vi "Fix BDPW Checksum.vi"(9 "Terminal Counts":T1, 10 "Only fix 3rd hash (F)":bool, 11 "Resources in":T2) -> (3 "Resources out":T2)   [LabVIEW 2018, in "Resource Manipulation.lvlib"]
uses:
  Resource Manipulation/Resource Array.ctl
  Resource Manipulation/Resource.ctl
  Resource Manipulation/Terminal Counts.ctl
  <userlib>/_OpenG.lib/md5/md5.llb/MD5 Message Digest (Binary String)__ogtk.vi
  Resource Manipulation/Find Resource by Type (String).vi
  Resource Manipulation.lvlib
panel:
  # "Thank you Thomas Zeugner! You saved me the trouble of figuring out how this checksum works. :)\nAdapted from https://github.com/tomsoftware/VI-Explorer/blob/master/php/clBDPW.php"
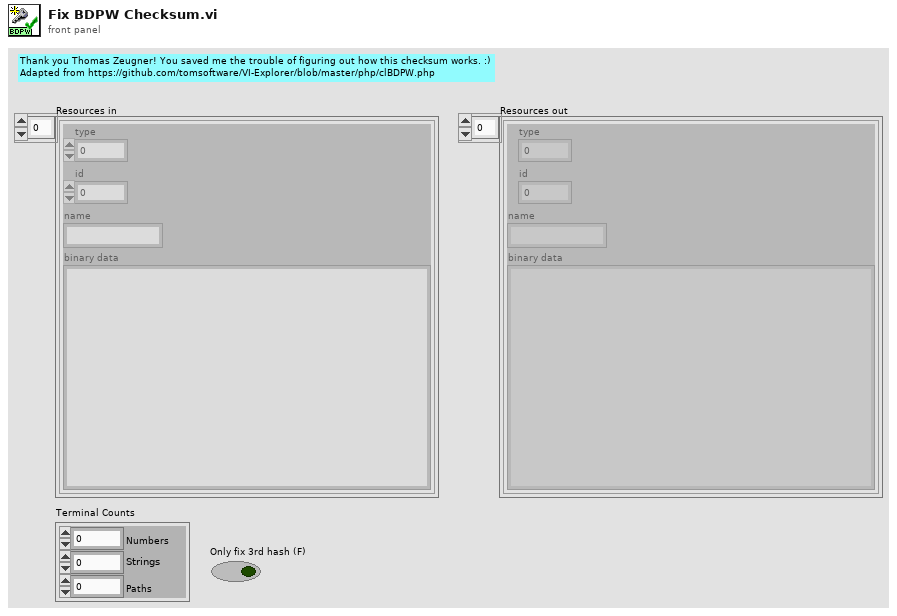
[diagram p1: front panel]
types:
  T1 = typedef "Resource Manipulation.lvlib/Terminal Counts.ctl" = cluster{"Numbers":u32, "Strings":u32, "Paths":u32}
  T2 = typedef "Resource Manipulation.lvlib/Resource Array.ctl" = T3[]
  T3 = typedef "Resource Manipulation.lvlib/Resource.ctl" = cluster{"type":u32, "id":i32, "name":string, "binary data":string}
  T4 = enum16{"big-endian, network order", "native, host order", "little-endian"}
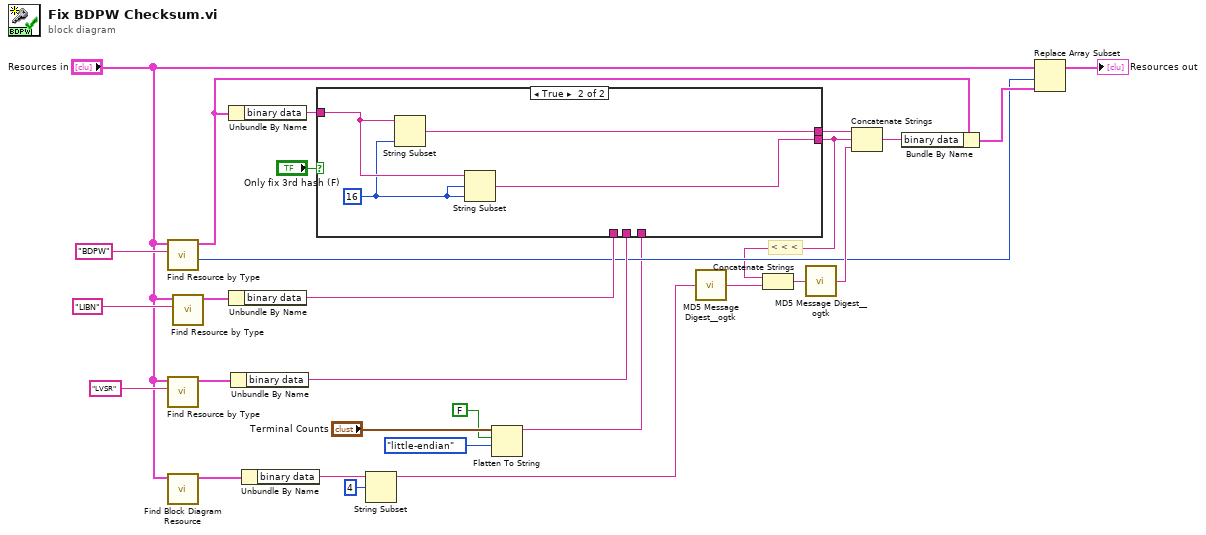
[diagram p0: block diagram]
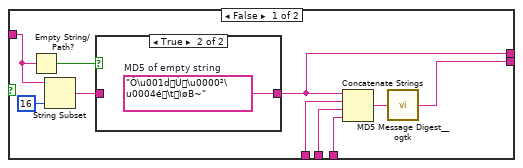
[diagram p2: hidden frame]
diagram:
  # "< < <"
  n1 = call-poly "Find Resource by Type.vi"("Resource Type"="BDPW", "Resources"="Resources in") -> ("Index"=w14:i32, "Resource"=w13:T3)  [unwired: 6 in, 2 out]
  n2 = call-poly "Find Resource by Type.vi"("Resource Type"="LVSR", "Resources"="Resources in") -> ("Resource"=w26:T3)  [unwired: 6 in, 3 out]
  n3 = call "Find Block Diagram Resource.vi"("Resources"="Resources in") -> ("Resource"=w10:T3)  [unwired: 8 in, 2 out]
  n4 = call-poly "Find Resource by Type.vi"("Resource Type"="LIBN", "Resources"="Resources in") -> ("Resource"=w27:T3)  [unwired: 6 in, 3 out]
  n5 = Unbundle By Name(w13) -> ("binary data"=w7:string)
  n6 = Unbundle By Name(w27) -> ("binary data"=w25:string)
  n7 = Unbundle By Name(w26) -> ("binary data"=w24:string)
  n8 = Unbundle By Name(w10) -> ("binary data"=w18:string)
  n9 = String Subset(string=w18, offset (0)=4) -> (substring=w16:string)  [unwired: 1 in]
  n10 = Flatten To String(anything="Terminal Counts", prepend array or string size? (T)=FALSE, byte order (0:big-endian, network order)=T4."little-endian") -> (data string=w3:string)  [unwired: 1 in, 2 out]
  n11 = case shown="True" "Only fix 3rd hash (F)" {
    tunnel: w25 -> [w37 _]
    tunnel: w24 -> [w36 _]
    tunnel: w3 -> [w34 _]
    tunnel: [w33 w41] -> w6
    tunnel: [w32 w42] -> w8
    tunnel: w7 -> [w30 w44]
    frame False {
      n12 = Empty String/Path?(string/path=w30) -> (empty?=w29:bool)
      n13 = String Subset(string=w30, length (rest)=16 ("length (rest)")) -> (substring=w31:string)  [unwired: 1 in]
      n14 = case shown="True" w29 {
        tunnel: [w39 w40] -> w32
        tunnel: w31 -> [w39 _]
        frame False {
        }
        frame True {
          w40 = "Ô\u001dÙ\u0000²\u0004é\tìøB~"  # MD5 of empty string
        }
      }
      n15 = Concatenate Strings(w32, w37, w36, w34) -> (w35:string)
      n16 = call-poly <userlib>:"MD5 Message Digest__ogtk.vi"("Message"=w35) -> ("MD5 Message Digest"=w33:string)
    }
    frame True {
      w43 = 16 ("length (rest)")
      n17 = String Subset(string=w44, length (rest)=w43) -> (substring=w42:string)  [unwired: 1 in]
      n18 = String Subset(string=w44, offset (0)=w43, length (rest)=w43) -> (substring=w41:string)
    }
  }
  n19 = call-poly <userlib>:"MD5 Message Digest__ogtk.vi"("Message"=w16) -> ("MD5 Message Digest"=w17:string)
  n20 = Concatenate Strings(w6, w17) -> (w20:string)
  n21 = call-poly <userlib>:"MD5 Message Digest__ogtk.vi"("Message"=w20) -> ("MD5 Message Digest"=w19:string)
  n22 = Concatenate Strings(w8, w6, w19) -> (w23:string)
  n23 = Bundle By Name(cluster=w13, "binary data"=w23) -> (w22:T3)
  n24 = Replace Array Subset(array="Resources in", new element=w22, index=w14) -> (→"Resources out":T2)
